vi "Digital Write Multiple Channels.vi"(8 "error in (no error)":errorcluster, 9 "Values":bool[](array[boolean]), 10 "Indices":i32[](array[numeric]), 11 "NI-DAQ in":refnum<class "NI-DAQ.lvclass">) -> (0 "error out":errorcluster, 3 "NI-DAQ out":refnum<class "NI-DAQ.lvclass">)   [LabVIEW 2021, in "NI-DAQ.lvclass"]
uses:
  NI-DAQ.lvclass
  NI-DAQ.lvclass/NI-DAQ.ctl
  <vilib>/Utility/file.llb/Read Delimited Spreadsheet (string).vi
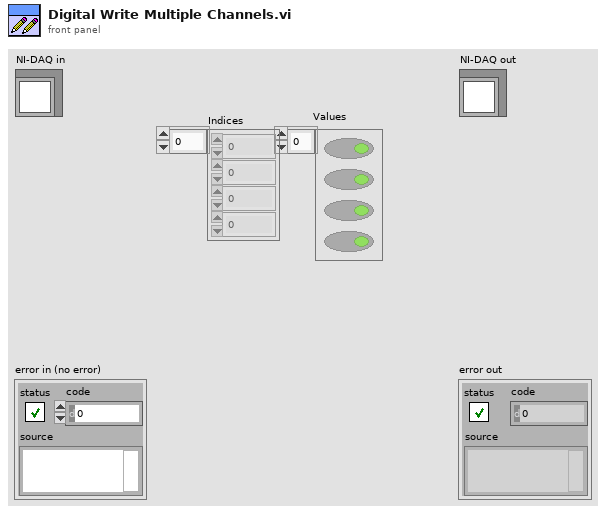
[diagram p1: front panel]
types:
  T1 = typedef "File Paths.ctl" = cluster{"Glue Pattern Folder":path, "Carrier Tray Folder":path, "Pick Up Tool Fixture Folder":path, "Components Folder":path, "Bellows Tool Offset.txt":path, "Pick Up Tool Offset.txt":path, "Dispense Tip Offset.txt":path, "Log Files":path, "Gantry Assembly Map.txt":path, "Syringe and offset map.txt":path, "Controllers Folder":path, "Local dbase config":path}
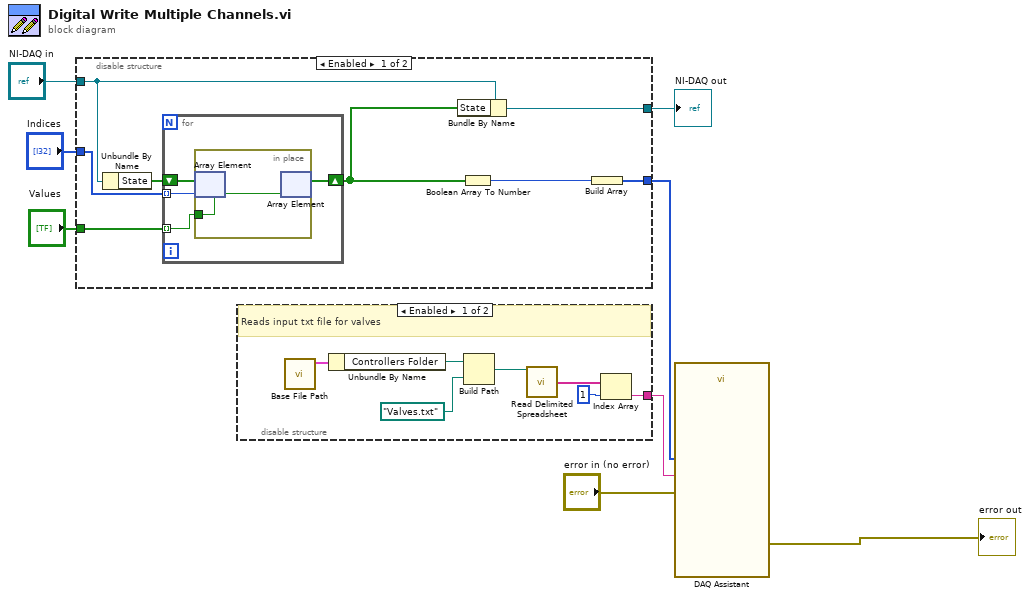
[diagram p0: block diagram]
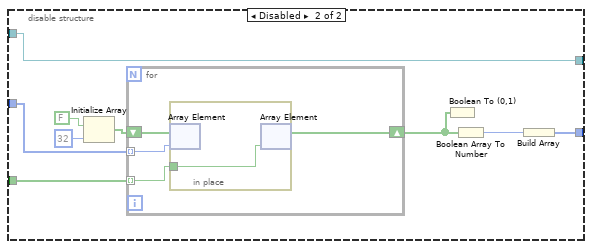
[diagram p3: hidden frame]
diagram:
  n1 = disable-structure shown="Enabled" {
    disable-tunnel: "NI-DAQ in" -> [w15 w30]
    disable-tunnel: [w14 w30] -> w7
    disable-tunnel: "Indices" -> [w11 w22]
    disable-tunnel: "Values" -> [w10 w23]
    disable-tunnel: [w9 w24] -> w3
    frame Enabled {
      n2 = Unbundle By Name(w15) -> ("State"=w13:bool[])
      n3 = for {
        tunnel: w10 -> [w20] mode=indexing
        tunnel: w11 -> [w19] mode=indexing
        shift-right: [w17] -> w12
        shift-left: w13 -> [w18]
        n4 = in-place {
          in-place-border: w20 -> [w21]
          n5 = in-place-array #1(w18, w19) -> ()  [unwired: 1 out]
          n6 = in-place-array #1(w21) -> (w17:bool[])  [unwired: 1 out]
        }
      }
      n7 = Bundle By Name(cluster=w15, "State"=w12) -> (w14:refnum<class "NI-DAQ.lvclass">)
      n8 = Boolean Array To Number(Boolean array=w12) -> (number=w16:u32)
      n9 = Build Array(w16) -> (w9:u32[])
    }
    frame Disabled {
      n10 = Initialize Array(FALSE, 32 ("dimension size")) -> (w29:bool[])
      n11 = for {
        tunnel: w22 -> [w34] mode=indexing
        tunnel: w23 -> [w33] mode=indexing
        shift-right: [w31] -> w26
        shift-left: w29 -> [w32]
        n12 = in-place {
          in-place-border: w33 -> [w35]
          n13 = in-place-array #2(w32, w34) -> ()  [unwired: 1 out]
          n14 = in-place-array #2(w35) -> (w31:bool[])  [unwired: 1 out]
        }
      }
      n15 = Boolean To (0,1)(Boolean=w26) -> ()  [unwired: 1 out]
      n16 = Boolean Array To Number(Boolean array=w26) -> (number=w25:u32)
      n17 = Build Array(w25) -> (w24:u32[])
    }
  }
  "NI-DAQ out" <- w7
  n18 = disable-structure shown="Enabled" {
    disable-tunnel: [w36 _] -> w1
    frame Enabled {
      # "Reads input txt file for valves"
      n19 = call "Base File Path.vi"() -> ("Paths Out"=w42:T1)  [unwired: 11 in]
      n20 = Unbundle By Name(w42) -> ("Controllers Folder"=w41:path)
      n21 = Build Path(base path=w41, name or relative path=path "Valves.txt") -> (appended path=w39:path)
      n22 = call-poly <vilib>:"Read Delimited Spreadsheet.vi"("file path (dialog if empty)"=w39) -> ("first row"=w38:string[])  [unwired: 9 in, 5 out]
      n23 = Index Array(array=w38, index=1 ("dimension size")) -> (element=w36:string)
    }
    frame Disabled {
    }
  }
  n24 = call "DAQ Assistant"("data"=w3, "error in"="error in (no error)", "device name"=w1) -> ("error out"=→"error out":errorcluster)  [unwired: 15 in, 1 out]
